vi "get led state.vi"(8 "error in (no error)":errorcluster, 11 "led":u32(ring) items=["GREEN", "RED"]) -> (0 "error out":errorcluster, 2 "LED On/Off":bool, 3 "function return":i32)   [LabVIEW 2014, in "libroboticscape.lvlib"]
doc: "int get_led_state(led_t led);"
uses:
  libroboticscape.lvlib
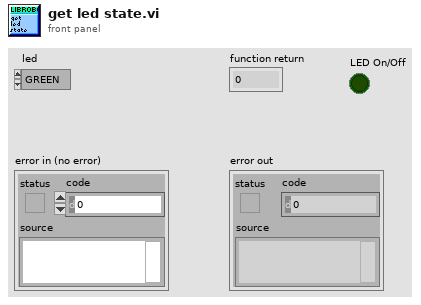
[diagram p1: front panel]
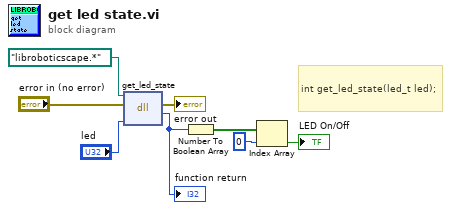
[diagram p0: block diagram]
diagram:
  # "int get_led_state(led_t led);"
  n1 = dll-call lib="C:/Users/ktalke/Documents/Robotics-Cape-Master-Jessie/Libroboticscape-Master-Jessie/libroboticscape.so" fn="get_led_state"(path in=path "libroboticscape.*", error in="error in (no error)", "led"="led") -> (error out=→"error out":errorcluster, "return type"=w4:i32)  [unwired: 2 in, 1 out]
  "function return" <- w4
  n2 = Number To Boolean Array(number=w4) -> (Boolean array=w3:bool[])
  n3 = Index Array(array=w3, index=0) -> (element=→"LED On/Off":bool)
